vi "send_readID_command.vi"() -> ()   [LabVIEW 2017]
panel:
  in  "数组 4":u32[](array[numeric])=[1, 1, 4]
  out "数组 3":string[](array[string])
  in  "数组 2":string[](array[string])=["shift:\u0005\u0000\u0000\u0000\u001f\u0000", "shift:\u0004\u0000\u0000\u0000\u0002\u0000", "shift: \u0000\u0000\u0000\u0000\u0000"]
  out "数据输出":string
  in  "数组":string[](array[string])=["shift:\u0005\u0000\u0000\u0000\u001f\u0000", "shift:\u0004\u0000\u0000\u0000\u0002\u0000", "shift: \u0000\u0000\u0000\u0000\u0000"]
  in  "服务器关闭":string="服务器VI关闭了连接。"
  in  "停止":bool
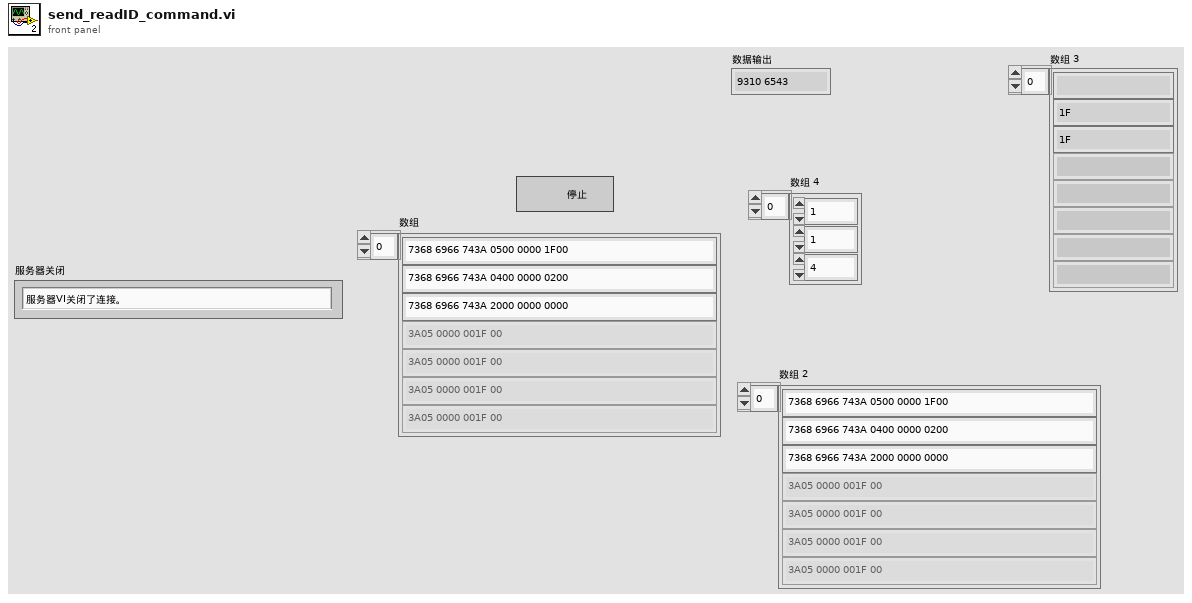
[diagram p1: front panel]
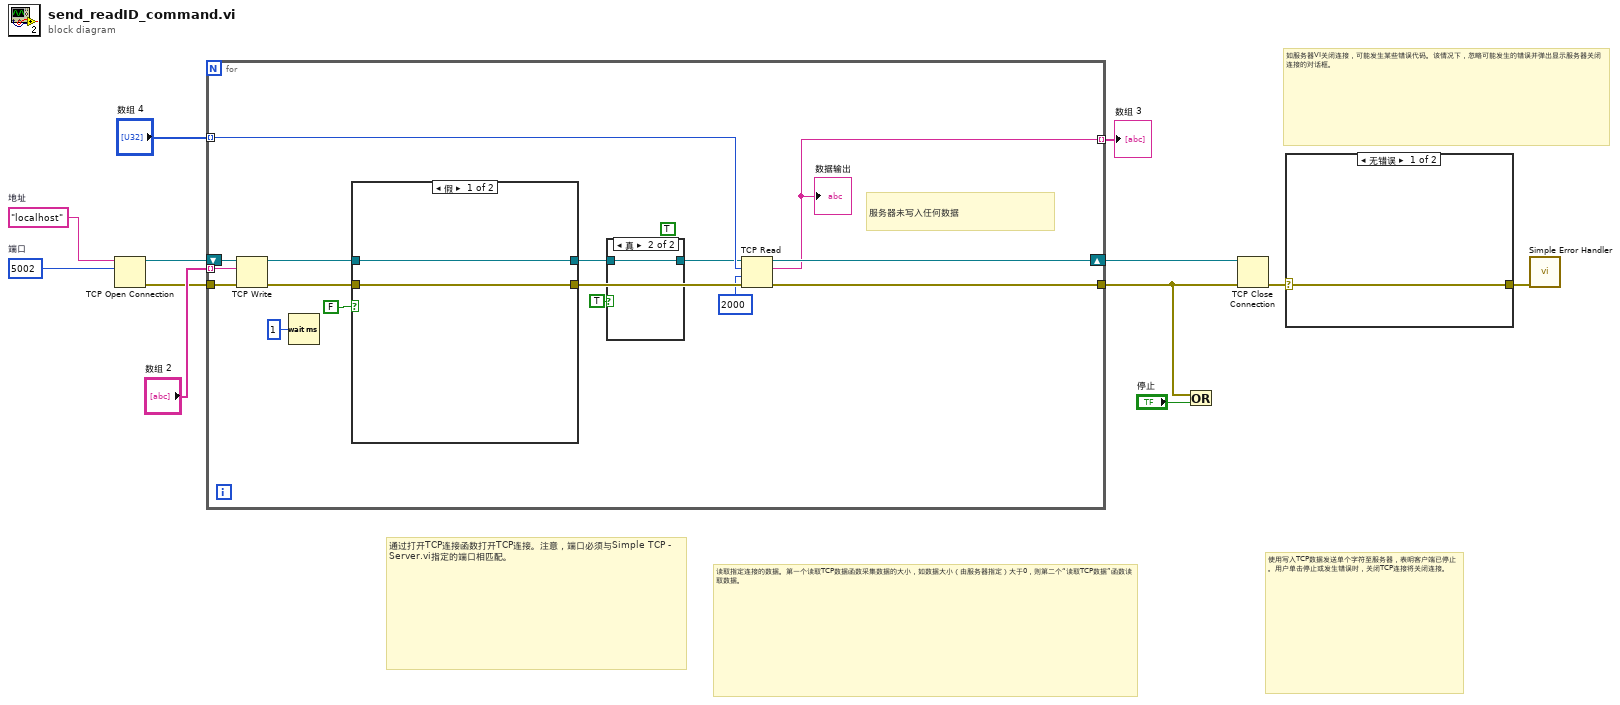
[diagram p0: block diagram]
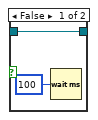
[diagram p2: hidden frame]
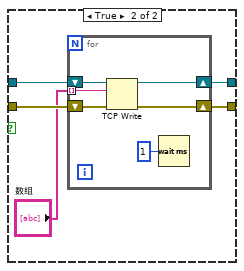
[diagram p3: hidden frame]
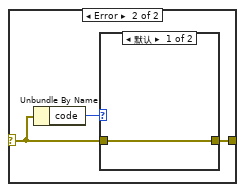
[diagram p4: hidden frame]
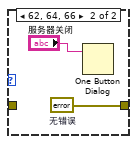
[diagram p5: hidden frame]
diagram:
  w9 = u16 5002  # 端口
  w10 = "localhost"  # 地址
  # "如服务器VI关闭连接，可能发生某些错误代码。该情况下，忽略可能发生的错误并弹出显示服务器关闭连接的对话框。"
  # "使用写入TCP数据发送单个字符至服务器，表明客户端已停止。用户单击停止或发生错误时，关闭TCP连接将关闭连接。"
  # "读取指定连接的数据。第一个读取TCP数据函数采集数据的大小，如数据大小（由服务器指定）大于0，则第二个“读取TCP数据”函数读取数据。"
  # "通过打开TCP连接函数打开TCP连接。注意，端口必须与Simple TCP - Server.vi指定的端口相匹配。"
  n1 = TCP Open Connection(address=w10, remote port or service name=w9) -> (connection ID=w7:refnum<k5>, error out=w6:errorcluster)  [unwired: 3 in]
  n2 = for {
    tunnel: "数组 2" -> [w26] mode=indexing
    shift-right: [w28] -> w2
    shift-left: w7 -> [w25]
    tunnel: [w17] -> w4 mode=indexing
    tunnel: w6 -> [w24]
    tunnel: [w27] -> w1
    tunnel: "数组 4" -> [w16] mode=indexing
    (unwired) TRUE
    # "服务器未写入任何数据"
    n3 = TCP Write(connection ID=w25, data in=w26, error in (no error)=w24) -> (connection ID out=w23:refnum<k5>, error out=w22:errorcluster)  [unwired: 1 in, 1 out]
    n4 = Wait (ms)(milliseconds to wait=u32 1) -> ()  [unwired: 1 out]
    n5 = case shown="假" FALSE {
      tunnel: w23 -> [w33 w38]
      tunnel: w22 -> [w32 w37]
      tunnel: [w33 w36] -> w15
      tunnel: [w32 w35] -> w21
      frame False {
      }
      frame True {
        n6 = for {
          shift-right: [w42] -> w36
          shift-left: w38 -> [w44]
          shift-right: [w41] -> w35
          shift-left: w37 -> [w43]
          tunnel: "数组" -> [w40] mode=indexing
          n7 = TCP Write(connection ID=w44, data in=w40, error in (no error)=w43) -> (connection ID out=w42:refnum<k5>, error out=w41:errorcluster)  [unwired: 1 in, 1 out]
          n8 = Wait (ms)(milliseconds to wait=u32 1) -> ()  [unwired: 1 out]
        }
      }
    }
    n9 = case shown="真" TRUE {
      tunnel: w15 -> [w30 w31]
      tunnel: [w30 w31] -> w14
      frame False {
        n10 = Wait (ms)(milliseconds to wait=u32 100) -> ()  [unwired: 1 out]
      }
      frame True {
      }
    }
    n11 = TCP Read(connection ID=w14, bytes to read=w16, error in (no error)=w21, 9:2000 ("timeout ms (25000)")) -> (connection ID out=w28:refnum<k5>, data out=w17:string, error out=w27:errorcluster)  [unwired: 1 in]
    "数据输出" <- w17
  }
  "数组 3" <- w4
  n12 = Or(x=w1, y="停止") -> ()  [unwired: 1 out]
  n13 = TCP Close Connection(connection ID=w2, error in (no error)=w1) -> (error out=w12:errorcluster)  [unwired: 1 in, 1 out]
  n14 = case shown="无错误" w12 {
    selector: w12 -> [w45 w47]
    tunnel: [w45 w46] -> w11
    frame No Error {
    }
    frame Error {
      n15 = Unbundle By Name(w47) -> ("code"=w48:i32)
      n16 = case shown="默认" w48 {
        tunnel: w47 -> [w49 _]
        tunnel: [w49 w51] -> w46
        frame Default {
        }
        frame 62, 64, 66 {
          w51 = errorcluster {"status"=FALSE, "code"=0, "source"=""}  # 无错误
          n17 = One Button Dialog(message="服务器关闭") -> ()  [unwired: 1 in, 1 out]
        }
      }
    }
  }
  n18 = call <vilib>:"Simple Error Handler.vi"("error in (no error)"=w11) -> ()  [unwired: 4 in, 5 out]
